vi "rasmy.vi"() -> ()   [LabVIEW 2026]
uses:
  <vilib>/addons/control/pid/pid.llb/PID Advanced (DBL).vi
  <vilib>/addons/control/pid/NI_PID_pid.lvlib
panel:
  in  "Output Valve 2":dbl(slide) scale=0.0..10.0
  in  "Output Valve 3":dbl(slide) scale=0.0..10.0
  in  "Output Valve 1":dbl(slide) scale=0.0..10.0
  out "LCV":dbl(knob) scale=0.0..100.0
  out "Waveform Chart":T1(graph)
  out "PV(OUTPUT)":dbl(slide) scale=0.0..100.0
  in  "PP":T2={"static gain"=2.5, "lag (s)"=2.5, "deadtime (s)"=0.001, "load"=0.0, "deadband"=0.0, "sensor noise"=0.0, "initial PV"=30.0, "plant noise"=0.0} {"plant noise" format="%.2f"; "initial PV" format="%.2f"; "sensor noise" format="%.2f"; "lag (s)" format="%.2f"; "deadtime (s)" format="%.2f"; "deadband" format="%.1f"; "load" format="%.2f"; "static gain" format="%.2f"}
  in  "PID gains":T3={"proportional gain (Kc)"=1.0, "integral time (Ti, min)"=0.01, "derivative time (Td, min)"=0.0} {"derivative time (Td, min)" format="%.3f"; "integral time (Ti, min)" format="%.3f"; "proportional gain (Kc)" format="%.3f"}
  in  "SP":dbl(slide) scale=0.0..100.0
  in  "auto":bool=TRUE
  in  "LCV":dbl format="%.2f"
  in  "stop":bool
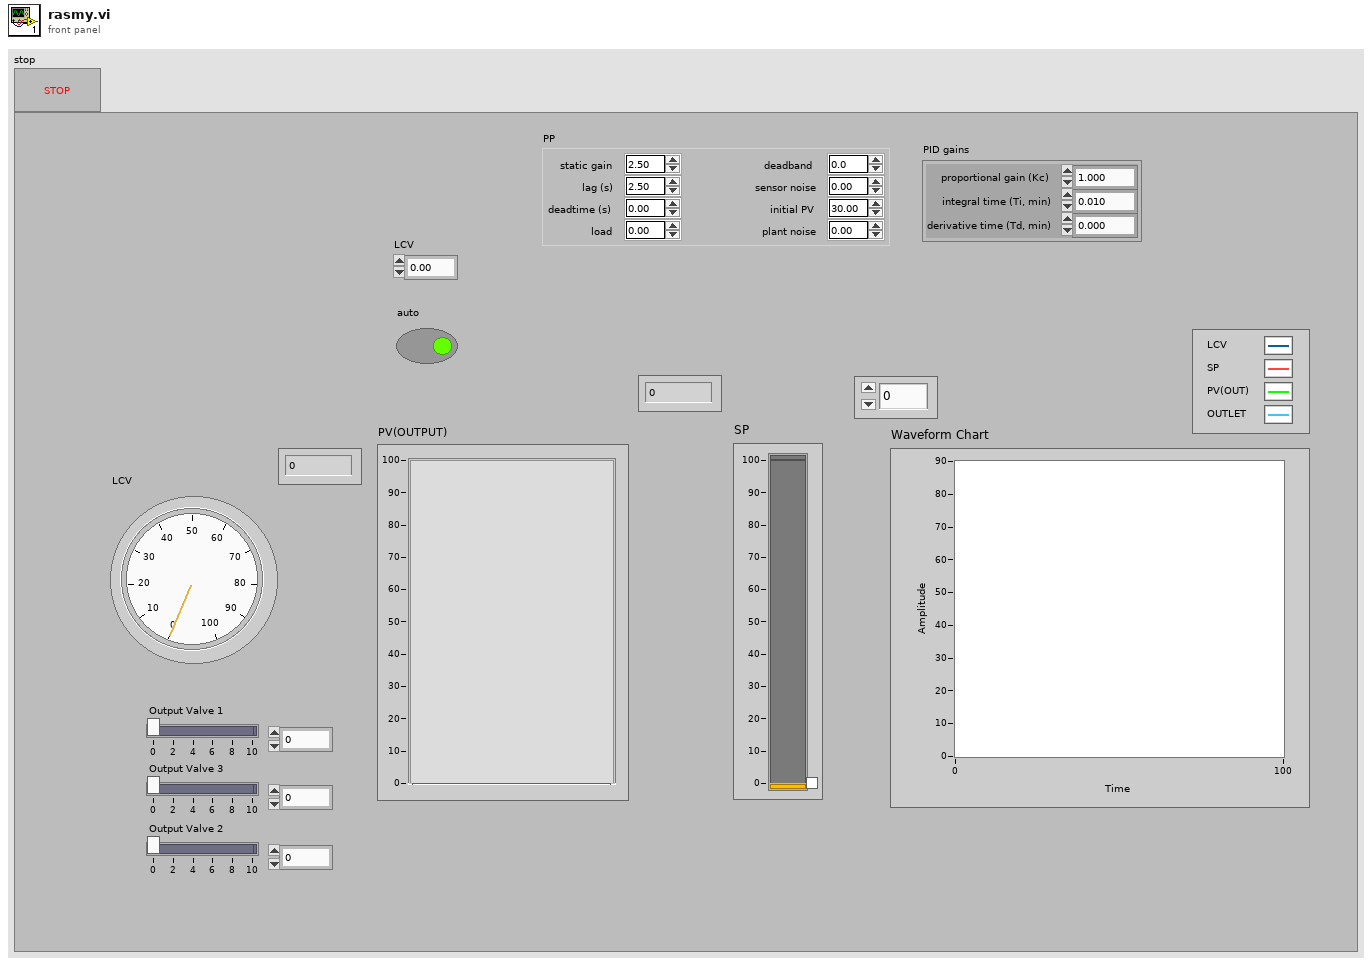
[diagram p1: front panel]
types:
  T1 = cluster{"output":dbl, "SP":dbl, "Plant Output":dbl, dbl}
  T2 = cluster{"static gain":dbl, "lag (s)":dbl, "deadtime (s)":dbl, "load":dbl, "deadband":dbl, "sensor noise":dbl, "initial PV":dbl, "plant noise":dbl}
  T3 = cluster{"proportional gain (Kc)":dbl, "integral time (Ti, min)":dbl, "derivative time (Td, min)":dbl}
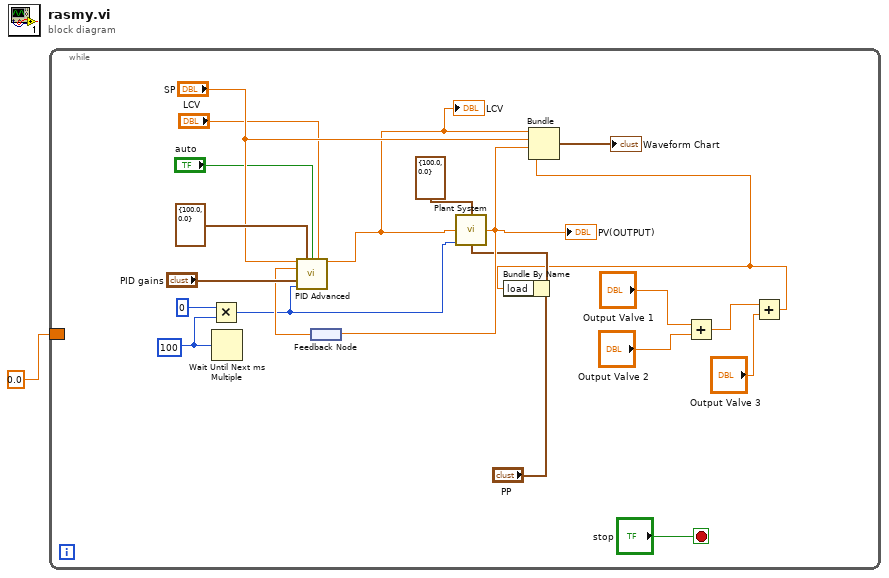
[diagram p0: block diagram]
diagram:
  n1 = while {
    border: 0.0 ("Plant Output") -> [_]
    stop <- "stop" stop-if-true
    w20 = u32 100 ("millisecond multiple")
    n2 = Multiply(x=u32 0, y=w20) -> (x*y=w13:u32)
    n3 = Wait Until Next ms Multiple(millisecond multiple=w20) -> ()  [unwired: 1 out]
    n4 = feedback #1() -> (w17:dbl)
    n5 = call-poly <vilib>:"PID Advanced.vi"("setpoint"="SP", "output range"=cluster{"output high":dbl, "output low":dbl} {"output high"=100.0, "output low"=0.0}, "auto? (T)"="auto", "manual control"="LCV", "process variable"=w17, "PID gains"="PID gains", "dt (s)"=w13) -> ("output"=w14:dbl)  [unwired: 7 in, 1 out]
    "LCV" <- w14
    n6 = Add(x="Output Valve 1", y="Output Valve 2") -> (x+y=w6:dbl)
    n7 = Add(x=w6, y="Output Valve 3") -> (x+y=w4:dbl)
    n8 = Bundle By Name(cluster="PP", "load"=w4) -> (w9:T2)
    n9 = call "Plant System.vi"("output saturation range"=cluster{"output high":dbl, "output low":dbl} {"output high"=100.0, "output low"=0.0}, "Plant Input"=w14, "dt (s)"=w13, "process parameters"=w9) -> ("Plant Output"=w11:dbl)  [unwired: 11 in]
    "PV(OUTPUT)" <- w11
    n10 = feedback-in #1(w11) -> ()
    n11 = Bundle("output"=w14, "SP"="SP", "Plant Output"=w11, w4) -> (→"Waveform Chart":T1)  [unwired: 1 in]
  }
